vi "Update Series View.vi"(10 "Intensity Series":variant[](array[variant]), 11 "Series Graph in":refnum<class "Graph with Series View.lvclass">) -> (3 "Series Graph out":refnum<class "Graph with Series View.lvclass">)   [LabVIEW 2023, in "Graph with Series View.lvclass"]
uses:
  Graph with Series View.lvclass
  Graph with Series View.lvclass/Graph with Series View.ctl
  Base Graph/Base Graph.lvclass
  D:/git/Lock-In-Thermography-Graphs/source/Detail Graph/Graph with Section Views.lvclass
  D:/git/Lock-In-Thermography-Graphs/source/Base Graph/Base Graph.lvclass
  D:/git/Lock-In-Thermography-Graphs/source/Series Graph/Graph with Series View.lvclass
panel:
  in  "Image #":u32
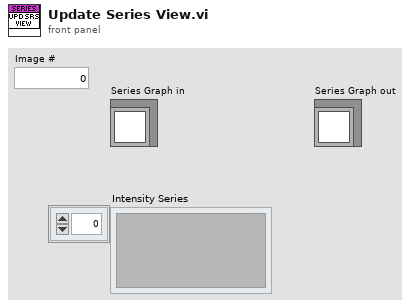
[diagram p1: front panel]
types:
  T1 = typedef "LVPointDoubleTypeDef.ctl" = cluster{"X":dbl, "Y":dbl}
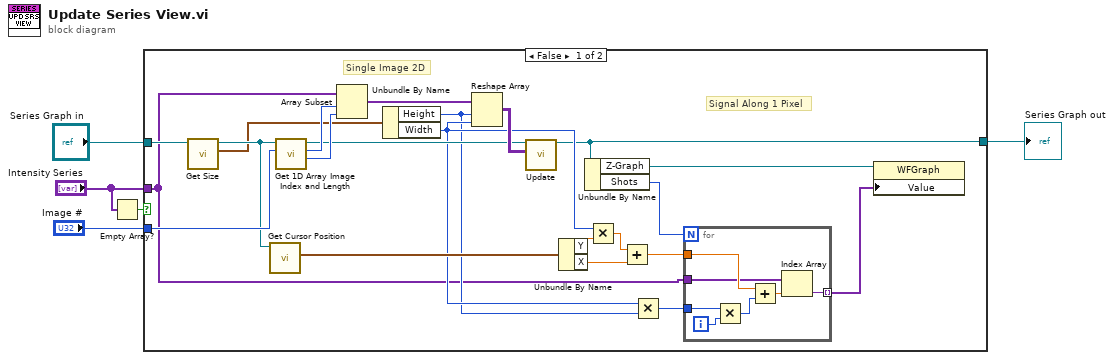
[diagram p0: block diagram]
diagram:
  n1 = Empty Array?(array="Intensity Series") -> (empty?=w1:bool)
  n2 = case shown="False" w1 {
    tunnel: [w8 w35] -> w5
    tunnel: "Series Graph in" -> [w14 w35]
    tunnel: "Image #" -> [w19 _]
    tunnel: "Intensity Series" -> [w6 _]
    frame False {
      # "Signal Along 1 Pixel"
      # "Single Image 2D"
      n3 = call "Get Size.vi"("Base Graph in"=w14) -> ("Sizes"=w12:cluster{"Height":u32, "Width":u32}, "Base Graph out"=w13:refnum<class "Graph with Series View.lvclass">)  [unwired: 9 in]
      n4 = call "Get Cursor Position.vi"("Base Graph in"=w13) -> ("Cursor Position"=w20:T1)  [unwired: 9 in, 1 out]
      n5 = call "Get 1D Array Image Index and Length.vi"("# Image"=w19, "Series Graph in"=w13) -> ("Image Length"=w16:u32, "Image Index"=w17:u32, "Series Graph out"=w11:refnum<class "Graph with Series View.lvclass">)  [unwired: 7 in]
      n6 = Array Subset(array=w6, index=w17, length=w16) -> (w18:variant[])
      n7 = Unbundle By Name(w12) -> ("Height"=w9:u32, "Width"=w10:u32)
      n8 = Reshape Array(w18, w9, w10) -> (w15:variant[][])
      n9 = call-dynamic "Update.vi"("Image"=w15, "Detail Graph in"=w11) -> ("Detail Graph out"=w8:refnum<class "Graph with Series View.lvclass">)  [unwired: 9 in]
      n10 = Unbundle By Name(w20) -> ("Y"=w25:dbl, "X"=w26:dbl)
      n11 = Unbundle By Name(w8) -> ("Z-Graph"=w22:refnum<vi>, "Shots"=w23:u32)
      n12 = Multiply(x=w10, y=w25) -> (x*y=w24:dbl)
      n13 = Add(x=w24, y=w26) -> (x+y=w7:dbl)
      n14 = Multiply(x=w10, y=w9) -> (x*y=w21:u32)
      n15 = for {
        N: w23 -> [_]
        tunnel: w6 -> [w29]
        tunnel: w21 -> [w33]
        tunnel: w7 -> [w30]
        tunnel: [w28] -> w27 mode=indexing
        i -> [w34]
        n16 = Multiply(x=w33, y=w34) -> (x*y=w31:u32)
        n17 = Add(x=w30, y=w31) -> (x+y=w32:dbl)
        n18 = Index Array(array=w29, index=w32) -> (element=w28:variant)
      }
      n19 = property class="WFGraph"(reference=w22, "Value"=w27) -> ()  [unwired: 1 in, 2 out]
    }
    frame True {
    }
  }
  "Series Graph out" <- w5
